vi "CE Measure for SS.vi"(5 "SS data directory":path, 6 "AC Source":T2, 7 "before SS? (T)":bool=TRUE, 8 "error in (no error)":errorcluster, 9 "PJVS":T5 {"NPL bias source"."DataSocketCluster"."TimeStamp" format="%.2f"}, 10 "CE measurement":T1 {"Switch position" format="%#_3p"; "Record lengths (multiples of periods)" format="%#_3p"; "Sampling frequencies (Hz)" format="%#_3p"; "Signal amplitudes (V)" format="%#_3p"; "Signal frequencies (Hz)" format="%#_3p"}, 11 "Common properties":T4={"Measurement status ref"=refnum, "TWM Status ref"=refnum, "Abort ref"=refnum, "Skip waiting ref"=refnum, "GNU Octave path"=path "C:/Program Files/GNU Octave/Octave-6.2.0/mingw64/bin", "TWM+QWTB path"=path "C:/Users/labina/Desktop/TWM-1.8.7.0-full/octprog", "lvlib path"=path "D:/martin/WAC/WACsw - github/control_software/Filter function meter/external libraries/GOLPI 0.7.3.1 source distribution LV 20.0 32 bit/lv_proc.dll", "TWM pipe"="\\\\.\\pipe\\TWM:server", "PJVS status ref"=refnum, "WAC path"=path ""}) -> (0 "error out":errorcluster, 1 "PJVS setup out":T5 {"NPL bias source"."DataSocketCluster"."TimeStamp" format="%.2f"}, 2 "CE measurement out":T1={"Signal frequencies (Hz)"=[1000.0], "Signal amplitudes (V)"=[0.707], "Sampling frequencies (Hz)"=[10000000.0], "Record lengths (multiples of periods)"=[10000.0], "TWM data root directory"=path "", "TWM mreasurements directories"=[], "Calculate RMS from samples"=FALSE, "RMS algorithm"="TWM-WFFT", "Settle down after AC source change (s)"=1.0, "Skip PJVS setup"=FALSE, "Measurement template file"=path "", "Row of START keyword"=0, "Row of STOP keyword"=0, "Measurement template line"=[], "Switch position"=[10000.0], "FR fit mat file"=path "", "Recalculate-skip already calculated"=FALSE} {"Switch position" format="%#_3p"; "Record lengths (multiples of periods)" format="%#_3p"; "Sampling frequencies (Hz)" format="%#_3p"; "Signal amplitudes (V)" format="%#_3p"; "Signal frequencies (Hz)" format="%#_3p"})   [LabVIEW 2020]
uses:
  Type definitions/CE measurement.ctl
  General PJVS driver/Type definitions/PJVS.ctl
  General PJVS driver/Type definitions/PJVS Type.ctl
  external libraries/acsvcontrol-driver/Public/Type Definitions/Timeouts.ctl
  external libraries/JV modified NPL Bias source/DataSocketCluster external.ctl
  Utilities/Type definitions/Common properties.ctl
  General AC source/Type definitions/AC Source.ctl
  General AC source/Type definitions/AC Source type.ctl
  external libraries/acsvcontrol-driver/ACSVcontrol-driver.lvlib
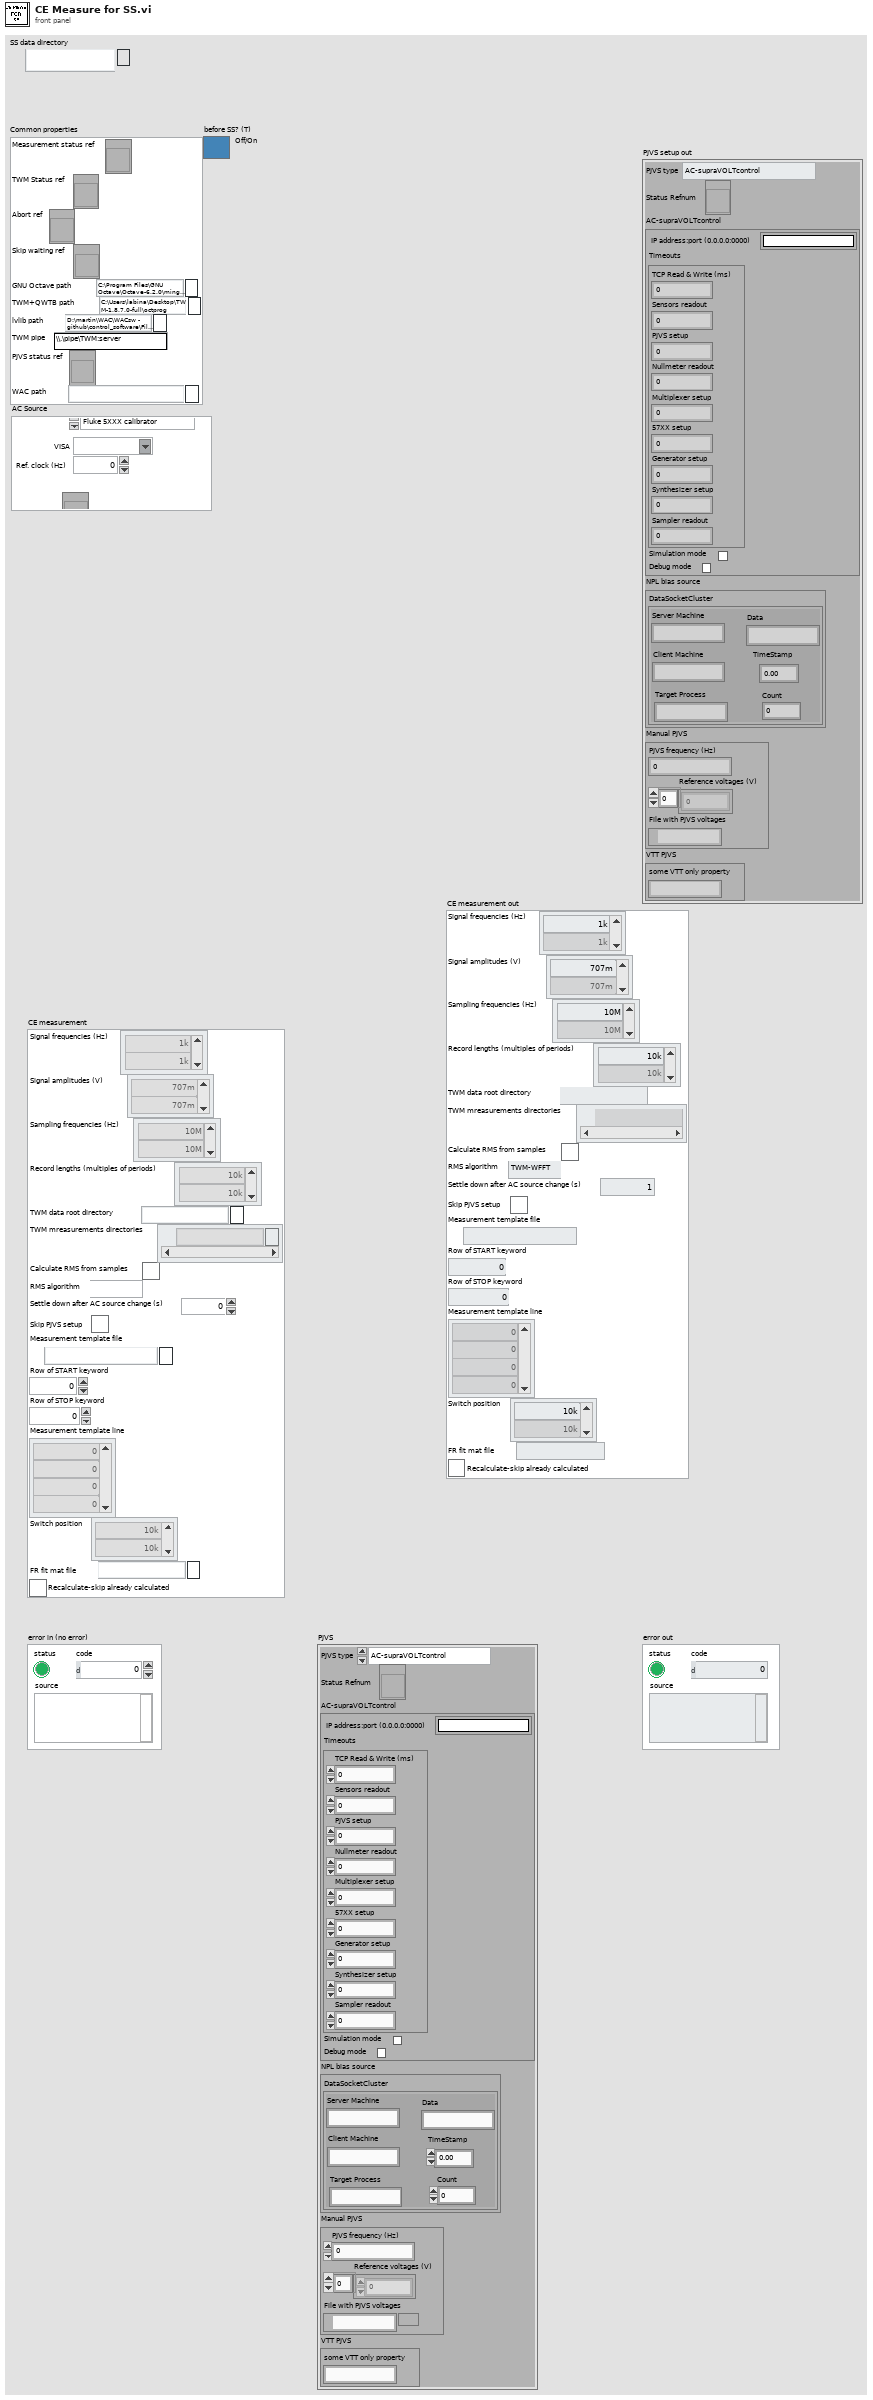
[diagram p1: front panel]
types:
  T1 = typedef "CE measurement.ctl" = cluster{"Signal frequencies (Hz)":dbl[], "Signal amplitudes (V)":dbl[], "Sampling frequencies (Hz)":dbl[], "Record lengths (multiples of periods)":dbl[], "TWM data root directory":path, "TWM mreasurements directories":path[], "Calculate RMS from samples":bool, "RMS algorithm":string, "Settle down after AC source change (s)":dbl, "Skip PJVS setup":bool, "Measurement template file":path, "Row of START keyword":i32, "Row of STOP keyword":i32, "Measurement template line":i32[], "Switch position":dbl[], "FR fit mat file":path, "Recalculate-skip already calculated":bool}
  T2 = typedef "AC Source.ctl" = cluster{"AC Source type":T3, "VISA":refnum<visa-resource-name>, "Ref. clock (Hz)":dbl, "status ref":refnum<vi>}
  T3 = typedef "AC Source type.ctl" = enum16{"Fluke 5XXX calibrator", "Tektronix AFG3000 series", "dummy", "Agilent 331xxA to 332xxA", "Agilent 335xxA to 336xxA"}
  T4 = typedef "Common properties.ctl" = cluster{"Measurement status ref":refnum<vi>, "TWM Status ref":refnum<vi>, "Abort ref":refnum<vi>, "Skip waiting ref":refnum<vi>, "GNU Octave path":path, "TWM+QWTB path":path, "lvlib path":path, "TWM pipe":string, "PJVS status ref":refnum<vi>, "WAC path":path}
  T5 = typedef "PJVS.ctl" = cluster{"PJVS type":T6, "Status Refnum":refnum<vi>, "AC-supraVOLTcontrol":cluster{"IP address:port (0.0.0.0:0000)":string, "Timeouts":T7, "Simulation mode":bool, "Debug mode":bool}, "NPL bias source":cluster{"DataSocketCluster":T8}, "Manual PJVS":cluster{"PJVS frequency (Hz)":dbl, "Reference voltages (V)":dbl[], "File with PJVS voltages":path}, "VTT PJVS":cluster{"some VTT only property":string}}
  T6 = typedef "PJVS Type.ctl" = enum16{"AC-supraVOLTcontrol", "JV modified NPL bias control", "Manual PJVS", "VTT PJVS"}
  T7 = typedef "ACSVcontrol-driver.lvlib/Timeouts.ctl" = cluster{"TCP Read & Write (ms)":i32, "Sensors readout":i32, "PJVS setup":i32, "Nullmeter readout":i32, "Multiplexer setup":i32, "57XX setup":i32, "Generator setup":i32, "Synthesizer setup":i32, "Sampler readout":i32}
  T8 = typedef "DataSocketCluster external.ctl" = cluster{"Server Machine":string, "Client Machine":string, "Data":string, "TimeStamp":dbl, "Count":i32, "Target Process":string}
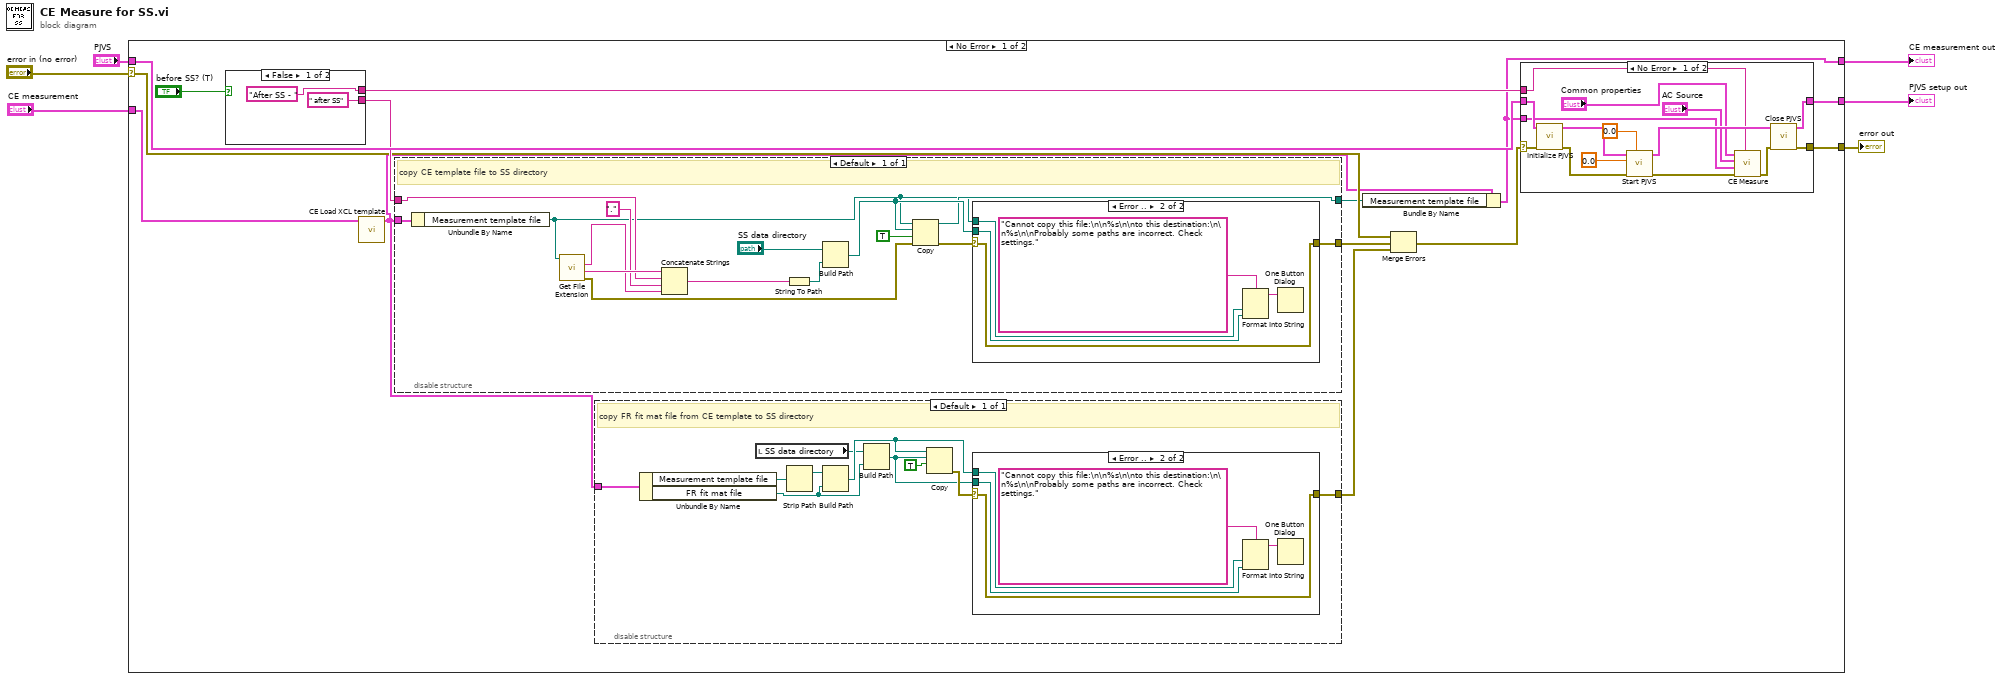
[diagram p0: block diagram]
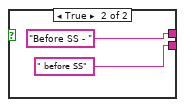
[diagram p5: hidden frame]
diagram:
  n1 = case shown="No Error" "error in (no error)" {
    selector: "error in (no error)" -> [w14 w80]
    tunnel: [w20 w80] -> w6
    tunnel: [w19 w81] -> w5
    tunnel: "PJVS" -> [w18 w81]
    tunnel: [w10 w79] -> w2
    tunnel: "CE measurement" -> [w9 w79]
    frame No Error {
      n2 = case shown="False" "before SS? (T)" {
        tunnel: ["After SS - " ("name suffix ()") "Before SS - " ("name suffix ()")] -> w16
        tunnel: [" after SS" ("string") " before SS" ("string")] -> w15
        frame False {
        }
        frame True {
        }
      }
      n3 = call "CE Load XCL template.vi"("CE measurement"=w9) -> ("CE measurement out"=w7:T1)  [unwired: 10 in]
      n4 = disable-structure shown="Default" {
        disable-tunnel: w15 -> [w32]
        disable-tunnel: [w26] -> w13
        disable-tunnel: [w24] -> w11
        disable-tunnel: w7 -> [w22]
        frame Enabled {
          # "copy CE template file to SS directory"
          n5 = Unbundle By Name(w22) -> ("Measurement template file"=w21:path)
          n6 = call <vilib>:"Get File Extension.vi"("file"=w21) -> ("error out"=w28:errorcluster, "filename without extension"=w33:string, "lowercase file extension"=w29:string)  [unwired: 6 in, 2 out]
          n7 = Concatenate Strings(w33, w32, "." ("string"), w29) -> (w34:string)
          n8 = String To Path(string=w34) -> (path=w31:path)
          n9 = Build Path(base path="SS data directory", name or relative path=w31) -> (appended path=w25:path)
          n10 = Copy(8:w28, 9:TRUE ("overwrite (F)"), 10:w25, 11:w21) -> (0:w27:errorcluster, 3:w24:path)  [unwired: 1 in, 1 out]
          n11 = case shown="Error .." w27 {
            selector: w27 -> [w36 w39]
            tunnel: [w36 w39] -> w26
            tunnel: w21 -> [_ w38]
            tunnel: w25 -> [_ w37]
            frame No Error {
            }
            frame Error {
              n12 = Format Into String(format string="Cannot copy this file:\n\n%s\n\nto this destination:\n\n%s\n\nProbably some paths are incorrect. Check settings.", w38, w37) -> (resulting string=w40:string)  [unwired: 2 in, 1 out]
              n13 = One Button Dialog(message=w40) -> ()  [unwired: 1 in, 1 out]
            }
          }
        }
      }
      n14 = disable-structure shown="Default" {
        disable-tunnel: w7 -> [w51]
        disable-tunnel: [w49] -> w8
        frame Enabled {
          # "copy FR fit mat file from CE template to SS directory"
          n15 = Unbundle By Name(w51) -> ("Measurement template file"=w42:path, "FR fit mat file"=w47:path)
          n16 = local read "SS data directory"() -> (w43:path)
          n17 = Strip Path(path=w42) -> (stripped path=w44:path)  [unwired: 1 out]
          n18 = Build Path(base path=w44, name or relative path=w47) -> (appended path=w45:path)
          n19 = Build Path(base path=w43, name or relative path=w47) -> (appended path=w46:path)
          n20 = Copy(9:TRUE ("overwrite (F)"), 10:w46, 11:w45) -> (0:w48:errorcluster)  [unwired: 2 in, 2 out]
          n21 = case shown="Error .." w48 {
            selector: w48 -> [w52 w55]
            tunnel: [w52 w55] -> w49
            tunnel: w45 -> [_ w54]
            tunnel: w46 -> [_ w53]
            frame No Error {
            }
            frame Error {
              n22 = Format Into String(format string="Cannot copy this file:\n\n%s\n\nto this destination:\n\n%s\n\nProbably some paths are incorrect. Check settings.", w54, w53) -> (resulting string=w56:string)  [unwired: 2 in, 1 out]
              n23 = One Button Dialog(message=w56) -> ()  [unwired: 1 in, 1 out]
            }
          }
        }
      }
      n24 = Bundle By Name(cluster=w7, "Measurement template file"=w11) -> (w10:T1)
      n25 = Merge Errors(w14, w13, w8) -> (w12:errorcluster)
      n26 = case shown="No Error" w12 {
        selector: w12 -> [w59 w74]
        tunnel: [w72 w74] -> w20
        tunnel: [w68 w73] -> w19
        tunnel: w18 -> [w67 w73]
        tunnel: w16 -> [w60 _]
        tunnel: w10 -> [w58 _]
        frame No Error {
          n27 = call "Initialize PJVS.vi"("error in (no error)"=w59, "PJVS setup"=w67) -> ("error out"=w69:errorcluster, "PJVS setup out"=w65:T5)  [unwired: 8 in]
          n28 = call "Start PJVS.vi"("Requested PJVS frequency (Hz)"=0.0, "error in (pass through)"=w69, "Maximal signal amplitude (V)"=0.0, "PJVS setup"=w65) -> ("error out"=w70:errorcluster, "PJVS setup out"=w66:T5)  [unwired: 3 in, 3 out]
          n29 = call "CE Measure.vi"("figure prefix ()"=w60, "error in"=w70, "CE measurement"=w58, "AC Source"="AC Source", "Common properties"="Common properties") -> ("error out"=w71:errorcluster)  [unwired: 6 in]
          n30 = call "Close PJVS.vi"("error in (pass through)"=w71, "PJVS setup"=w66) -> ("error out"=w72:errorcluster, "PJVS setup out"=w68:T5)  [unwired: 8 in]
        }
        frame Error {
        }
      }
    }
    frame Error {
    }
  }
  "error out" <- w6
  "PJVS setup out" <- w5
  "CE measurement out" <- w2
